vi "New Bitmap Canvas.vi"(8 "error in (no error)":errorcluster, 11 "Size":cluster{"Width":u16, "Height":u16}) -> (0 "error out":errorcluster, 3 "Bitmap Canvas out":refnum<class "Bitmap Canvas.lvclass">)   [LabVIEW 2023, in "Font Glyph Drawer Interface.lvlib" / "Bitmap Canvas.lvclass"]
uses:
  Bitmap Canvas.lvclass
  Bitmap Canvas.lvclass/Bitmap Canvas.ctl
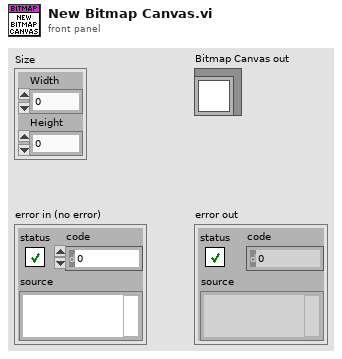
[diagram p1: front panel]
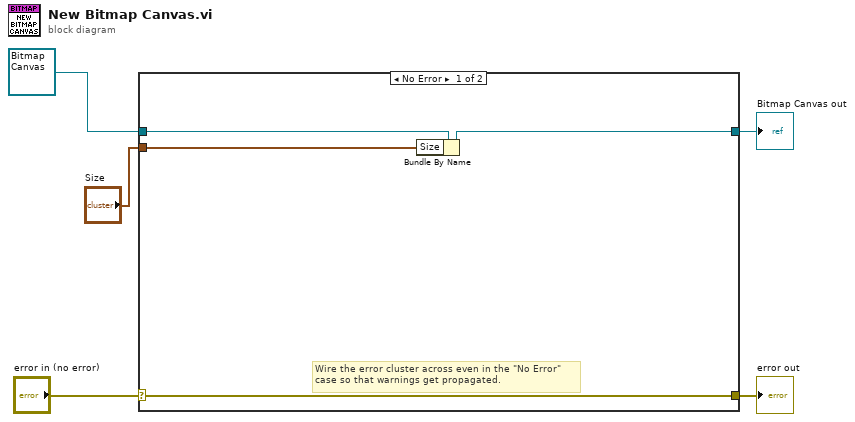
[diagram p0: block diagram]
diagram:
  n1 = case shown="No Error" "error in (no error)" {
    selector: "error in (no error)" -> [w8 w11]
    tunnel: [w8 w11] -> w4
    tunnel: [w7 w10] -> w2
    tunnel: refnum<class "Bitmap Canvas.lvclass"> refnum ("Bitmap Canvas in") -> [w9 w10]
    tunnel: "Size" -> [w6 _]
    frame No Error {
      # "Wire the error cluster across even in the \"No Error\"\ncase so that warnings get propagated."
      n2 = Bundle By Name(cluster=w9, "Size"=w6) -> (w7:refnum<class "Bitmap Canvas.lvclass">)
    }
    frame Error {
    }
  }
  "error out" <- w4
  "Bitmap Canvas out" <- w2
